vi "OE1022_Configure Sine Out.vi"(7 "OE1022_Configure Sine Out":T1={"Start Value(V)"=0.1, "Sine Output Amplitude (V)"=0.1, "Stop Valve(V)"=1.0, "Sine Step Valve(V)"=0.1, "Step Time(ms) "=1000, "Sine Step Percent(%)"=10.0, "SineOut Mode"=0, "Sine Run Mode"=0} {"Sine Run Mode" items=["Stop", "Single", "Loop"]; "SineOut Mode" items=["Fixed", "Linear", "Log"]; "Sine Step Percent(%)" min=0.0 max=100.0 format="%#.3g"; "Step Time(ms)" min=1 max=100000; "Sine Step Valve(V)" min=0.001 max=5.0 format="%#.3g"; "Stop Valve(V)" min=0.0001 max=5.0 format="%#.3g"; "Sine Output Amplitude (V)" min=0.0001 max=5.0 format="%#.3g"; "Start Value(V)" min=0.001 max=5.0 format="%#.3g"}, 8 "Error in (no error)":errorcluster caption="error out（no error）", 9 "Remote Mode":u16(ring) items=["USB"=0, "GPIB"=2], 11 "VISA resource name":refnum<visa-resource-name>) -> (0 "Error out":errorcluster caption="error out", 1 "Output String":string, 3 "VISA resource  out":refnum<visa-resource-name>)   [LabVIEW 2011]
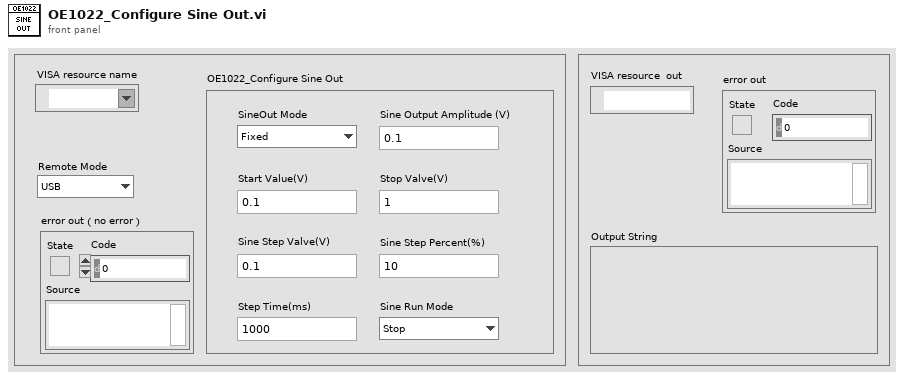
[diagram p1: front panel]
types:
  T1 = cluster{"Start Value(V)":dbl, "Sine Output Amplitude (V)":dbl, "Stop Valve(V)":dbl, "Sine Step Valve(V)":dbl, "Step Time(ms) ":u32, "Sine Step Percent(%)":dbl, "SineOut Mode":u8, "Sine Run Mode":u8}
  T2 = enum16{"ISRC", "IGND", "ICPL", "ILIN", "PHAS", "FMOD", "RSLP", "FREQ", "SWPT", "SLLM", "SULM", "SSLL", "SSLG", "STLM", "SWRM", "IRNG", "SENS", "RMOD", "OFLT", "OFSL", "SYNC", "DMOD", "HARM", "DARB", "SWVT", "SLVL", "SVLL", "SVUL", "SVSL", "SVSG", "SVTM", "SVRM", "RALL", "SNAP", "OUTP", "OAUX", "COUT", "CAUX", "COFP", "CEXP", "FPOP", "OEXP", "*IDN", "*RST", "OVLD", "INOV", "GNOV", "*PLL", "SSET", "RSET", "AGAN", "APHS", "ARSV", "ASCL", "EQCD", "EQCS", "SPED", "SRAT", "SLEN", "SSLE", "STRG", "SPRM", "STRD", "PAUS", "REST", "SPTS", "TRCA", "TEMP", "RSTU", "IHNZ", "DEQU", "SADD", "ARNG", "CSPE", "ISRCD", "IGNDD", "ICPLD", "ILIND", "PHASD", "FMODD", "RSLPD", "FREQD", "SWPTD", "SLLMD", "SULMD", "SSLLD", "SSLGD", "STLMD", "SWRMD", "SENSD", "RMODD", "OFLTD", "OFSLD", "SYNCD", "HARMD", "EQCDD", "EQCSD", "SNAPD", "OUTPD", "SWVTD", "SLVLD", "SVLLD", "SVULD", "SVSLD", "SVSGD", "SVTMD", "SVRMD", "SVDCD", "ARSVD", "AGAND", "APHSD", "ASCLD", "FPOPD", "CAUXD", "OEXPD", "SPEDD", "SRATD", "SLEND", "SSLED", "STRGD", "SPRMD", "STRDD", "PAUSD", "RESTD", "SPTSD", "TRCAD", "*IDND", "*RSTD", "INOVD", "GNOVD", "*PLLD", "SSETD", "RSETD"}
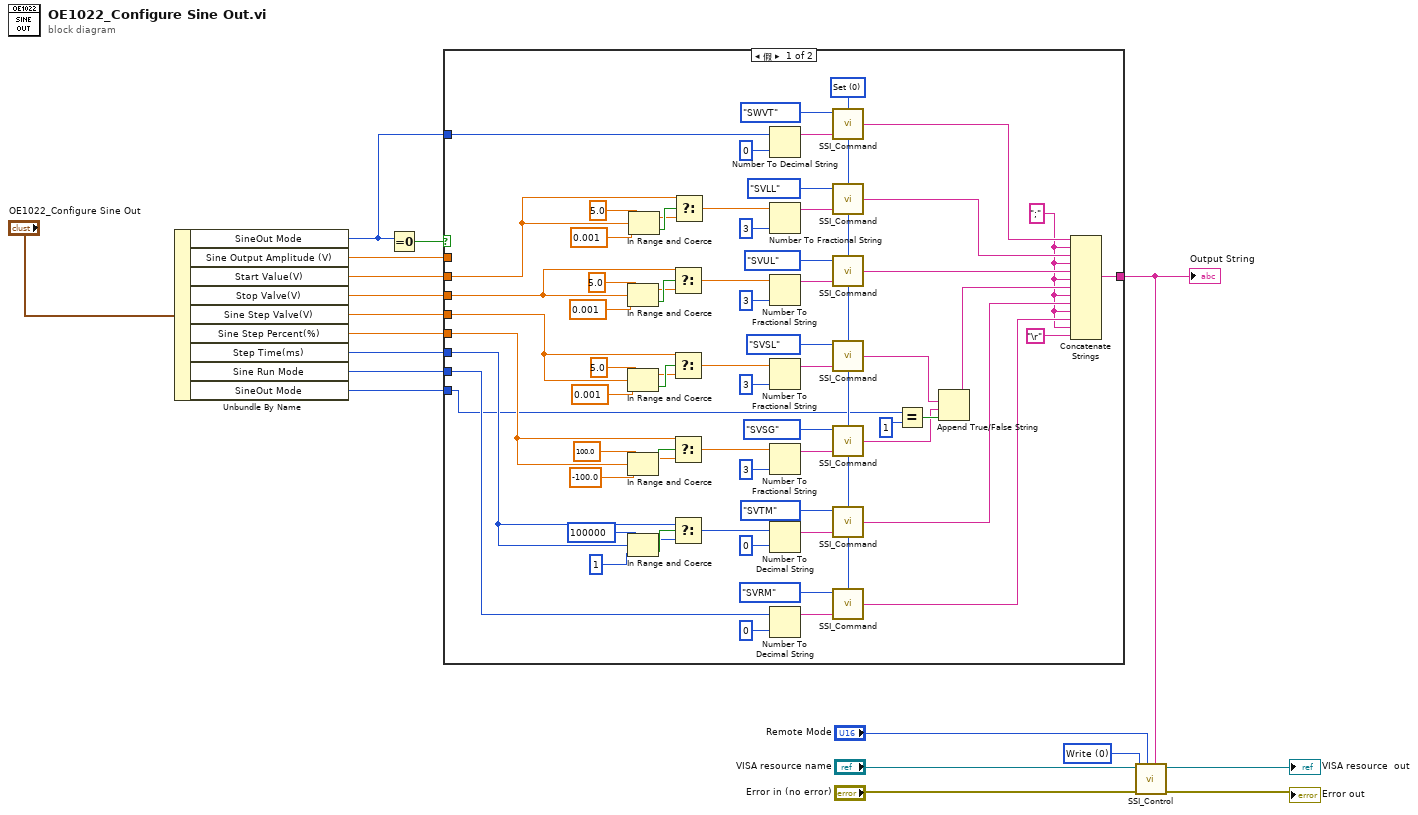
[diagram p0: block diagram]
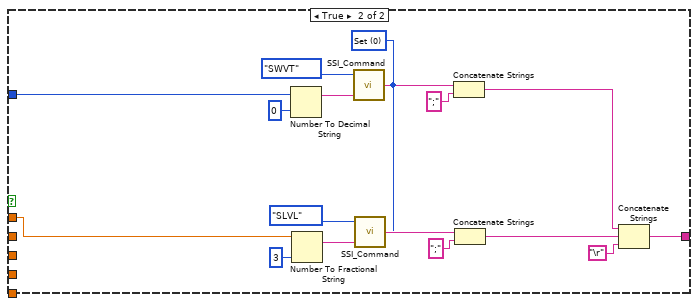
[diagram p2: hidden frame]
diagram:
  w17 = u16 0 items=["Write", "Read"] ("Control")
  n1 = Unbundle By Name("OE1022_Configure Sine Out") -> ("SineOut Mode"=w2:u8, "Sine Output Amplitude (V)"=w1:dbl, "Start Value(V)"=w10:dbl, "Stop Valve(V)"=w9:dbl, "Sine Step Valve(V)"=w8:dbl, "Sine Step Percent(%)"=w7:dbl, "Step Time(ms)"=w6:u32, "Sine Run Mode"=w5:u8, "SineOut Mode"=w3:u8)
  n2 = Equal To 0?(x=w2) -> (x = 0?=w11:bool)
  n3 = case shown="假" w11 {
    tunnel: [w43 w88] -> w4
    tunnel: w10 -> [w22 _]
    tunnel: w2 -> [w59 w94]
    tunnel: w9 -> [w23 _]
    tunnel: w8 -> [w35 _]
    tunnel: w7 -> [w53 _]
    tunnel: w6 -> [w52 _]
    tunnel: w5 -> [w40 _]
    tunnel: w3 -> [w20 _]
    tunnel: w1 -> [_ w87]
    frame False {
      w41 = ";"
      w55 = u16 0 items=["Set", "Query"] ("Opera")
      n4 = In Range and Coerce(upper limit=5.0 ("上限"), x=w23, lower limit=0.001 ("下限")) -> (coerced(x)=w33:dbl, In Range?=w34:bool)
      n5 = In Range and Coerce(upper limit=5.0 ("上限"), x=w35, lower limit=0.001 ("下限")) -> (coerced(x)=w38:dbl, In Range?=w39:bool)
      n6 = In Range and Coerce(upper limit=100.0 ("上限"), x=w53, lower limit=-100.0 ("下限")) -> (coerced(x)=w62:dbl, In Range?=w63:bool)
      n7 = In Range and Coerce(upper limit=u32 100000 ("上限"), x=w52, lower limit=u32 1 ("下限")) -> (coerced(x)=w66:u32, In Range?=w67:bool)
      n8 = In Range and Coerce(upper limit=5.0 ("上限"), x=w22, lower limit=0.001 ("下限")) -> (coerced(x)=w27:dbl, In Range?=w28:bool)
      n9 = Select(t=w23, s=w34, f=w33) -> (s? t:f=w30:dbl)
      n10 = Select(t=w35, s=w39, f=w38) -> (s? t:f=w29:dbl)
      n11 = Select(t=w53, s=w63, f=w62) -> (s? t:f=w19:dbl)
      n12 = Select(t=w52, s=w67, f=w66) -> (s? t:f=w54:u32)
      n13 = Select(t=w22, s=w28, f=w27) -> (s? t:f=w24:dbl)
      n14 = Number To Decimal String(number=w59, width (-)=i16 0 ("精度(6)")) -> (decimal integer string=w81:string)
      n15 = Number To Fractional String(number=w24, precision (6)=i16 3 ("精度(6)")) -> (F-format string=w78:string)  [unwired: 2 in]
      n16 = Number To Fractional String(number=w30, precision (6)=i16 3 ("精度(6)")) -> (F-format string=w75:string)  [unwired: 2 in]
      n17 = Number To Fractional String(number=w29, precision (6)=i16 3 ("精度(6)")) -> (F-format string=w72:string)  [unwired: 2 in]
      n18 = Number To Fractional String(number=w19, precision (6)=i16 3 ("精度(6)")) -> (F-format string=w69:string)  [unwired: 2 in]
      n19 = Number To Decimal String(number=w54, width (-)=i16 0 ("精度(6)")) -> (decimal integer string=w84:string)
      n20 = Number To Decimal String(number=w40, width (-)=i16 0 ("精度(6)")) -> (decimal integer string=w57:string)
      n21 = call "SSI_Command.vi"("Opera"=w55, "Paramter"=w81, "Command Type"=T2."SWVT") -> ("Output string"=w49:string)  [unwired: 1 in]
      n22 = call "SSI_Command.vi"("Opera"=w55, "Paramter"=w78, "Command Type"=T2."SVLL") -> ("Output string"=w48:string)  [unwired: 1 in]
      n23 = call "SSI_Command.vi"("Opera"=w55, "Paramter"=w75, "Command Type"=T2."SVUL") -> ("Output string"=w47:string)  [unwired: 1 in]
      n24 = call "SSI_Command.vi"("Opera"=w55, "Paramter"=w72, "Command Type"=T2."SVSL") -> ("Output string"=w50:string)  [unwired: 1 in]
      n25 = call "SSI_Command.vi"("Opera"=w55, "Paramter"=w69, "Command Type"=T2."SVSG") -> ("Output string"=w51:string)  [unwired: 1 in]
      n26 = call "SSI_Command.vi"("Opera"=w55, "Paramter"=w84, "Command Type"=T2."SVTM") -> ("Output string"=w45:string)  [unwired: 1 in]
      n27 = call "SSI_Command.vi"("Opera"=w55, "Paramter"=w57, "Command Type"=T2."SVRM") -> ("Output string"=w44:string)  [unwired: 1 in]
      n28 = Equal?(x=w20, y=u8 1 ("x")) -> (x = y?=w86:bool)
      n29 = Append True/False String(1:w86, 2:w51, 3:w50) -> (0:w46:string)  [unwired: 1 in]
      n30 = Concatenate Strings(w49, w41, w48, w41, w47, w41, w46, w41, w45, w41, w44, w41, "\r") -> (w43:string)
    }
    frame True {
      w95 = u16 0 items=["Set", "Query"] ("Opera")
      n31 = Number To Decimal String(number=w94, width (-)=i16 0 ("宽度(-)")) -> (decimal integer string=w97:string)
      n32 = Number To Fractional String(number=w87, precision (6)=i16 3 ("宽度(-)")) -> (F-format string=w101:string)  [unwired: 2 in]
      n33 = call "SSI_Command.vi"("Opera"=w95, "Paramter"=w97, "Command Type"=T2."SWVT") -> ("Output string"=w96:string)  [unwired: 1 in]
      n34 = call "SSI_Command.vi"("Opera"=w95, "Paramter"=w101, "Command Type"=T2."SLVL") -> ("Output string"=w100:string)  [unwired: 1 in]
      n35 = Concatenate Strings(w96, ";" ("替换字符串(\"\")")) -> (w89:string)
      n36 = Concatenate Strings(w100, ";" ("替换字符串(\"\")")) -> (w91:string)
      n37 = Concatenate Strings(w89, w91, "\r") -> (w88:string)
    }
  }
  "Output String" <- w4
  n38 = call "SSI_Control.vi"("Write Buffer"=w4, "Remote Mode"="Remote Mode", "Error in (no error)"="Error in (no error)", "Control"=w17, "VISA resource name"="VISA resource name") -> ("Error out"=→"Error out":errorcluster, "VISA resource  out"=→"VISA resource  out":refnum<visa-resource-name>)  [unwired: 3 in, 2 out]
